vi "niUSRP Tx Continuous Lab copy.vi"() -> ()   [LabVIEW 2014]
uses:
  <instrlib>/niUSRP/niUSRP Write Tx Data (CDB WDT).vi
panel:
  out "Waveform Graph":dbl[](graph)
  in  "Stop Button":bool
  out "IQ Plot":waveform(dbl)[](graph)
  in  "device name":refnum<k15>="192.168.10.2"
  out "Error Out":errorcluster
  in  "active antenna":string="TX/RX"
  out "Gain [dB] (actual)":dbl format="%#.6p"
  out "Carrier Frequency \n[Hz] (actual)":dbl=2450000000.0 format="%#.6p"
  out "IQ Sampling\nRate [s/sec] (actual)":dbl=10000000.0 format="%#.6p"
  in  "Gain [dB]":dbl format="%#.6p"
  in  "Carrier\nFrequency [Hz]":dbl=915000000.0 format="%#.6p"
  in  "IQ Sampling\nRate [s/sec]":dbl=10000000.0 format="%#.6p"
  # "IQ Transmitter"
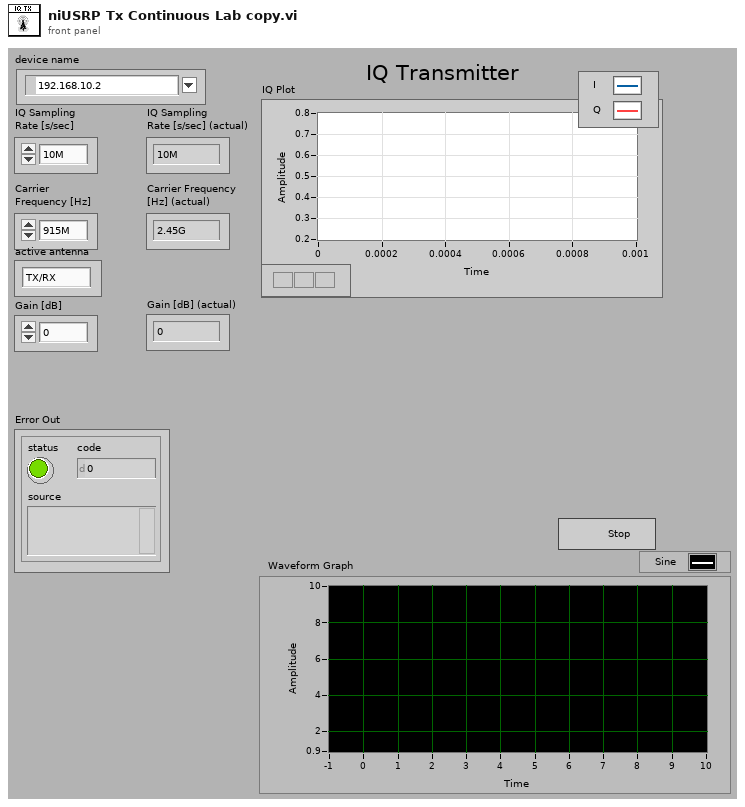
[diagram p1: front panel]
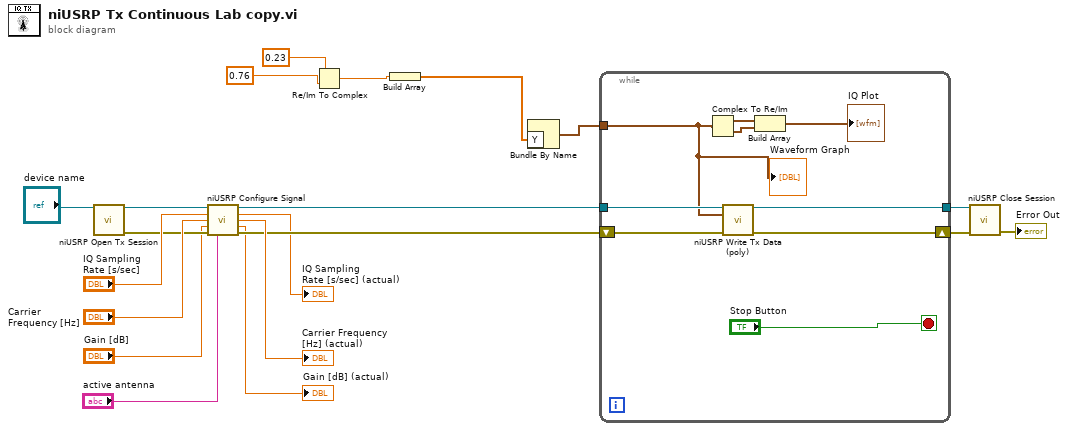
[diagram p0: block diagram]
diagram:
  n1 = call <instrlib>:"niUSRP Open Tx Session.vi"("device names"="device name") -> ("session handle out"=w20:refnum<k15>, "error out"=w17:errorcluster)  [unwired: 13 in]
  n2 = call <instrlib>:"niUSRP Configure Signal.vi"("session handle"=w20, "IQ rate"="IQ Sampling\nRate [s/sec]", "carrier frequency"="Carrier\nFrequency [Hz]", "gain"="Gain [dB]", "error in (no error)"=w17, "active antenna"="active antenna") -> ("session handle out"=w15:refnum<k15>, "coerced IQ rate"=→"IQ Sampling\nRate [s/sec] (actual)":dbl, "coerced carrier frequency"=→"Carrier Frequency \n[Hz] (actual)":dbl, "coerced gain"=→"Gain [dB] (actual)":dbl, "error out"=w14:errorcluster)  [unwired: 5 in]
  n3 = Re/Im To Complex(1:0.76, 2:0.23) -> (0:w3:cdb)
  n4 = Build Array(w3) -> (w4:cdb[])
  n5 = Bundle By Name("Y"=w4) -> (w5:waveform(cdb))  [unwired: 1 in]
  n6 = while {
    tunnel: w15 -> [w29]
    tunnel: [w27] -> w13
    shift-right: [w26] -> w12
    shift-left: w14 -> [w28]
    tunnel: w5 -> [w21]
    stop <- "Stop Button" stop-if-true
    n7 = Complex To Re/Im(x + iy=w21) -> (x=w24:waveform(dbl), y=w25:waveform(dbl))
    n8 = call-poly <instrlib>:"niUSRP Write Tx Data (poly).vi"("session handle"=w29, "data"=w21, "error in (no error)"=w28) -> ("session handle out"=w27:refnum<k15>, "error out"=w26:errorcluster)  [unwired: 11 in]
    n9 = Build Array(w24, w25) -> (→"IQ Plot":waveform(dbl)[])
    "Waveform Graph" <- w21
  }
  n10 = call <instrlib>:"niUSRP Close Session.vi"("session handle"=w13, "error in (no error)"=w12) -> ("error out"=→"Error Out":errorcluster)  [unwired: 13 in]
